vi "--lv_icon_editor--vi_tree.vi"   [LabVIEW 2021]
uses:
  <vilib>/LabVIEW Icon API/lv_icon/lv_icon.lvlib
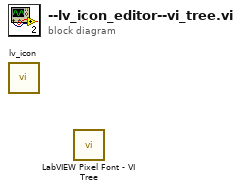
[diagram p0: block diagram]
diagram:
  n1 = call <resource>:"lv_icon.vi"() -> ()  [unwired: 9 in, 3 out]
  n2 = call <vilib>:"LabVIEW Pixel Font - VI Tree.vi"() -> ()  [unwired: 12 in]
